vi "labview_sessions_generate.vi"(4 "pswd":string, 5 "ip":string, 6 "user":string, 9 "Numeric":dbl, 11 "Path":path) -> (2 "Session Generator Output":string, 7 "return code":i32, 8 "error":string)   [LabVIEW 2015]
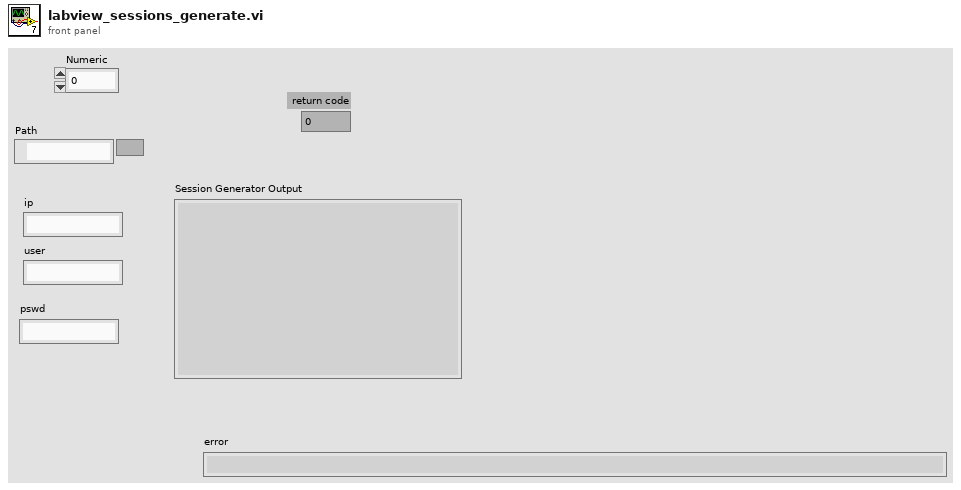
[diagram p1: front panel]
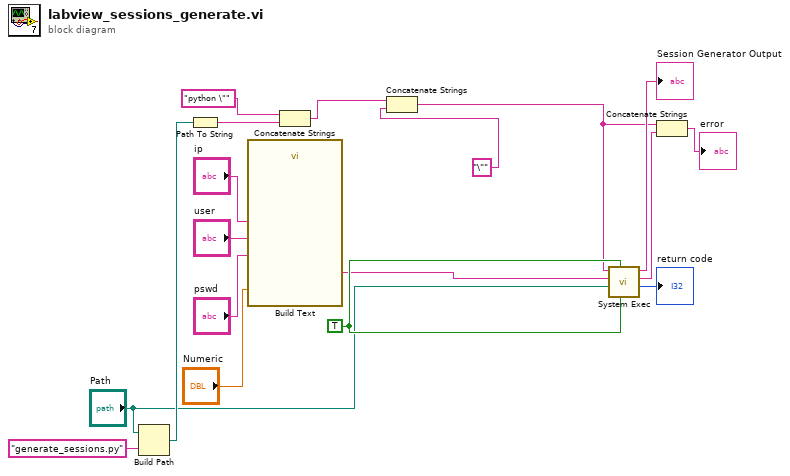
[diagram p0: block diagram]
diagram:
  w18 = TRUE
  n1 = Build Path(base path="Path", name or relative path="generate_sessions.py") -> (appended path=w15:path)
  n2 = Path To String(path=w15) -> (string=w17:string)
  n3 = call "Build Text"("error"="Numeric", "ip"="ip", "user"="user", "password"="pswd") -> ("Result"=w8:string)  [unwired: 10 in, 1 out]
  n4 = Concatenate Strings("python \"", w17) -> (w3:string)
  n5 = Concatenate Strings(w3, "\"") -> (w1:string)
  n6 = call <vilib>:"System Exec.vi"("run minimized? (F)"=w18, "wait until completion? (T)"=w18, "working directory"="Path", "standard input"=w8, "command line"=w1) -> ("return code"=→"return code":i32, "standard error"=w4:string, "standard output"=→"Session Generator Output":string)  [unwired: 3 in, 1 out]
  n7 = Concatenate Strings(w1, w4) -> (→"error":string)
